vi "Return SysCfg Session.vi"(8 "error in":errorcluster, 10 "SysCfg Session":refnum<k21>, 11 "Controller in":refnum<class "Controller.lvclass">) -> (0 "error out":errorcluster, 3 "Controller out":refnum<class "Controller.lvclass">)   [LabVIEW 2015, in "SMI.lvlib" / "Controller.lvclass"]
uses:
  Controller.lvclass
  SysCfg Device/SysCfg Device.lvclass/SysCfg Device.ctl
  SysCfg Device/Write SysCfg Session.vi
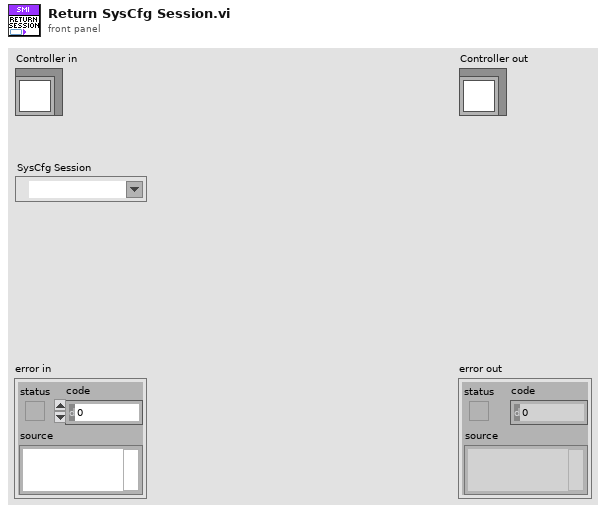
[diagram p1: front panel]
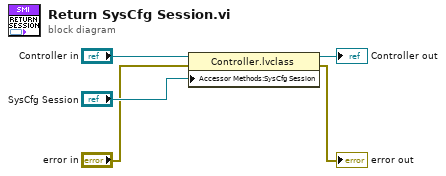
[diagram p0: block diagram]
diagram:
  n1 = property class="Controller.lvclass"(reference="Controller in", error in="error in", "Accessor Methods:SysCfg Session"="SysCfg Session") -> (reference out=→"Controller out":refnum<class "Controller.lvclass">, error out=→"error out":errorcluster)
